vi "stop.vi"(8 "error in (no error)":errorcluster, 11 "WriteSignalsGenericPlugin in":refnum<class "SignalWriterMH110203USBStepperMotor.lvclass">) -> (0 "error out":errorcluster, 3 "WriteSignalsGenericPlugin out":refnum<class "SignalWriterMH110203USBStepperMotor.lvclass">)   [LabVIEW 2010, in "SignalWriterMH110203USBStepperMotor.lvclass"]
uses:
  SignalWriterMH110203USBStepperMotor.lvclass
  SignalWriterMH110203USBStepperMotor.lvclass/SignalWriterMH110203USBStepperMotor.ctl
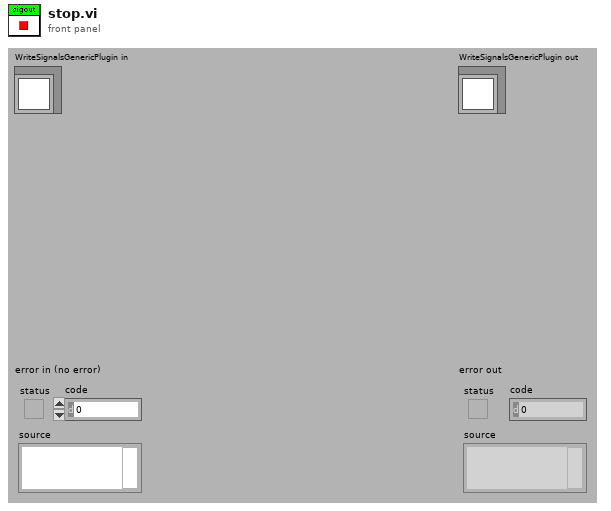
[diagram p1: front panel]
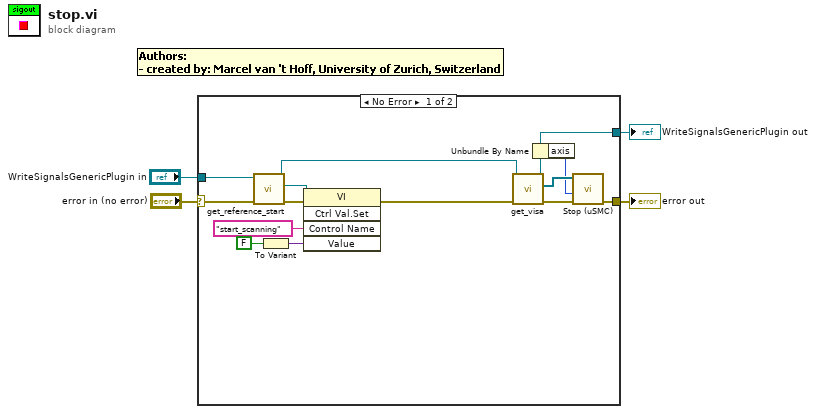
[diagram p0: block diagram]
diagram:
  n1 = case shown="No Error" "error in (no error)" {
    selector: "error in (no error)" -> [w12 w19]
    tunnel: "WriteSignalsGenericPlugin in" -> [w13 w20]
    tunnel: [w18 w19] -> w1
    tunnel: [w15 w20] -> w2
    frame No Error {
      n2 = call-dynamic "get_reference_start.vi"("error in (no error)"=w12, "SignalWriterMH110203USBStepperMotor in"=w13) -> ("error out"=w6:errorcluster, "vi reference"=w7:refnum<vi>, "SignalWriterMH110203USBStepperMotor out"=w5:refnum<class "SignalWriterMH110203USBStepperMotor.lvclass">)  [unwired: 7 in]
      n3 = To Variant(anything=FALSE) -> (Variant=w10:variant)
      n4 = invoke class="VI" method="Ctrl Val.Set"(reference=w7, error in=w6, "Control Name"="start_scanning", "Value"=w10) -> (error out=w11:errorcluster)  [unwired: 1 in, 4 out]
      n5 = call-dynamic "get_visa.vi"("error in (no error)"=w11, "SignalWriterMH110203USBStepperMotor in"=w5) -> ("error out"=w16:errorcluster, "visa array"=w17:refnum<visa-resource-name>[], "SignalWriterMH110203USBStepperMotor out"=w15:refnum<class "SignalWriterMH110203USBStepperMotor.lvclass">)  [unwired: 6 in, 1 out]
      n6 = Unbundle By Name(w15) -> ("axis"=w14:i32)
      n7 = call "Stop (uSMC).vi"("error in (no error)"=w16, "Index"=w14, "Visa array in"=w17) -> ("error out"=w18:errorcluster)  [unwired: 7 in, 1 out]
    }
    frame Error {
    }
  }
  "error out" <- w1
  "WriteSignalsGenericPlugin out" <- w2
